vi "motorRate TEST.vi"() -> ()   [LabVIEW 2019]
uses:
  <vilib>/rvi/Emulation/niFpgaGetClockAttributes.vi
  <vilib>/rvi/Emulation/niFpgaSctlEmulationGetInTimedLoop.vi
  <vilib>/rvi/Emulation/niFpgaEmulationReportErrorSimple.vi
  <vilib>/rvi/Emulation/niFpgaCriticalErrorInLSC.vi
panel:
  out "Time since last execution":u32
  in  "stop":bool
  out "Data Out":T1 {"ID" format="%x"}
  in  "Control Value":fxp<+/-,32,16>
  in  "ID":u32 format="%x"
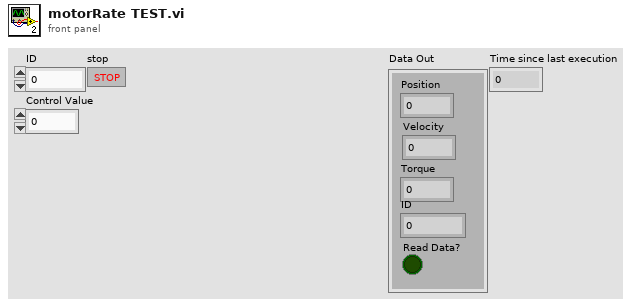
[diagram p1: front panel]
types:
  T1 = cluster{"Position":fxp<+/-,32,16>, "Velocity":fxp<+/-,32,16>, "Torque":fxp<+/-,32,16>, "ID":u32, "Read Data?":bool}
  T2 = typedef "SPI Config.ctl" = cluster{"MXP Port":enum16{"A", "B"}, "Device":enum16{"CAN", "ENC", "IMU1", "IMU2"}, "CPOL":bool}
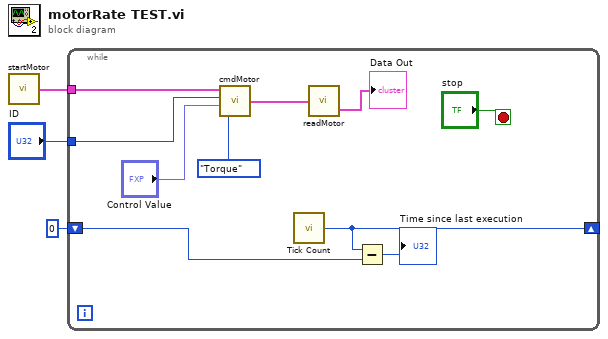
[diagram p0: block diagram]
diagram:
  n1 = call "startMotor.vi"() -> ("SPI Config Out"=w3:T2)  [unwired: 2 in]
  n2 = while {
    tunnel: w3 -> [w12]
    tunnel: "ID" -> [w11]
    shift-right: [w6] -> _
    shift-left: u32 0 ("Tick Count(uSec)") -> [w5]
    stop <- "stop" stop-if-true
    n3 = call "cmdMotor.vi"("Mode"=enum16{"Position", "Velocity", "Torque"}."Torque", "Control Value"="Control Value", "ID"=w11, "SPI Config In"=w12) -> ("SPI Config Out"=w13:T2)
    n4 = call "Tick Count"() -> ("Tick Count(uSec)"=w6:u32)
    n5 = call "readMotor.vi"("SPI Config In"=w13) -> ("Data Out"=→"Data Out":T1)  [unwired: 1 out]
    n6 = Subtract(x=w6, y=w5) -> (x-y=→"Time since last execution":u32)
  }
